vi "Save Errors Status.vi"(5 "Lot":string, 6 "Stress":string, 7 "Wafer":string, 8 "error in (no error)":errorcluster, 9 "File Name":string, 10 "Error Status":string, 11 "base path":path=path "C:/temp") -> (0 "error out":errorcluster)   [LabVIEW 2017]
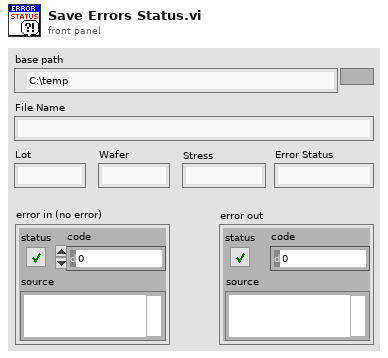
[diagram p1: front panel]
types:
  T1 = enum16{"open", "replace", "create", "open or create", "replace or create", "replace or create with confirmation"}
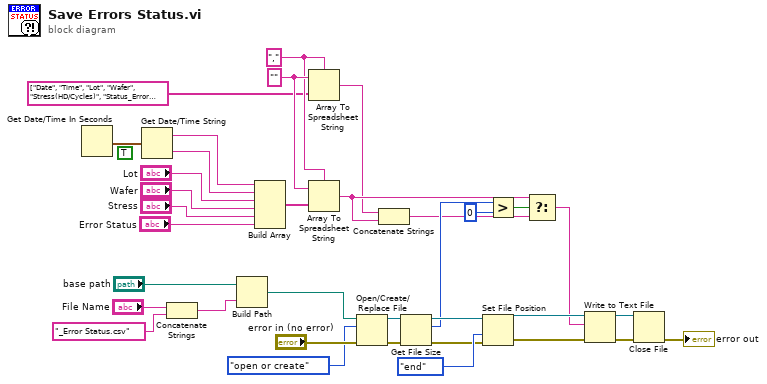
[diagram p0: block diagram]
diagram:
  (unwired) TRUE ("want seconds? (F)")
  w15 = "," ("delimiter (Tab)")
  w16 = "" ("format string")
  n1 = Get Date/Time In Seconds() -> (seconds since 1Jan1904=w8:timestamp)
  n2 = Get Date/Time String(seconds (now)=w8) -> (date string=w7:string, time string=w6:string)  [unwired: 2 in]
  n3 = Concatenate Strings("File Name", "_Error Status.csv" ("name or relative path")) -> (w34:string)
  n4 = Build Path(base path="base path", name or relative path=w34) -> (appended path=w19:path)
  n5 = Build Array(w7, w6, "Lot", "Wafer", "Stress", "Error Status") -> (w3:string[])
  n6 = Array To Spreadsheet String(delimiter (Tab)=w15, array=string[] ["Date", "Time", "Lot", "Wafer", "Stress(HD/Cycles)", "Status_Error Code"], 3:w16) -> (spreadsheet string=w12:string)
  n7 = Array To Spreadsheet String(delimiter (Tab)=w15, array=w3, 3:w16) -> (spreadsheet string=w14:string)
  n8 = Open/Create/Replace File(file path (use dialog)=w19, error in="error in (no error)", operation (0:open)=T1."open or create") -> (refnum out=w22:refnum<file>, error out=w21:errorcluster)  [unwired: 3 in, 1 out]
  n9 = Concatenate Strings(w12, w14) -> (w13:string)
  n10 = Get File Size(file=w22, error in=w21) -> (refnum out=w25:refnum<file>, size (in bytes)=w17:i64, 0:w23:errorcluster)
  n11 = Set File Position(refnum=w25, from (0:start)=enum16{"start", "end", "current"}."end", error in=w23) -> (refnum out=w27:refnum<file>, error out=w26:errorcluster)  [unwired: 1 in]
  n12 = Greater?(x=w17, y=i64 0) -> (0:w11:bool)
  n13 = Select(t=w14, s=w11, f=w13) -> (s? t:f=w10:string)
  n14 = Write to Text File(file (use dialog)=w27, text=w10, error in=w26) -> (refnum out=w31:refnum<file>, error out=w30:errorcluster)  [unwired: 1 in, 1 out]
  n15 = Close File(refnum=w31, error in=w30) -> (error out=→"error out":errorcluster)  [unwired: 1 out]
